vi "Add Alias_Alias and Alias Folder.vi"(8 "error in (no error)":errorcluster, 9 "Alias Settings":T1, 11 "SysDef Ref":T2) -> (0 "error out":errorcluster, 3 "SysDef Ref Out":T2)   [LabVIEW 2019, in "Simple SysDef API.lvlib"]
uses:
  <userlib>/SimpleSysDef/Simple SysDef API.lvlib
  <userlib>/SimpleSysDef/_SubVIs/System Definition Reference.ctl
  NationalInstruments.VeriStand.SystemDefinitionAPI
  <userlib>/SimpleSysDef/_SubVIs/Add Alias_Alias Settings.ctl
  <userlib>/SimpleSysDef/_SubVIs/Add Folder_Settings.ctl
  <userlib>/SimpleSysDef/_SubVIs/Add Alias Folder.vi
  <userlib>/SimpleSysDef/_SubVIs/Add Alias.vi
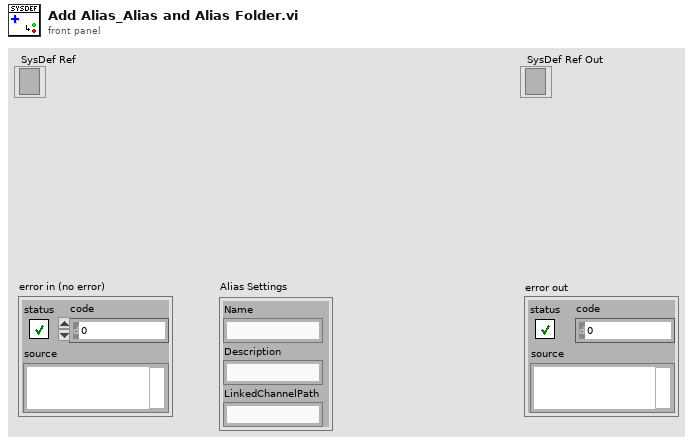
[diagram p1: front panel]
types:
  T1 = typedef "Simple SysDef API.lvlib/Add Alias_Alias Settings.ctl" = cluster{"Name":string, "Description":string, "LinkedChannelPath":string}
  T2 = typedef "Simple SysDef API.lvlib/System Definition Reference.ctl" = refnum<k24>
  T3 = typedef "Simple SysDef API.lvlib/Add Folder_Settings.ctl" = cluster{"Name":string, "Description":string}
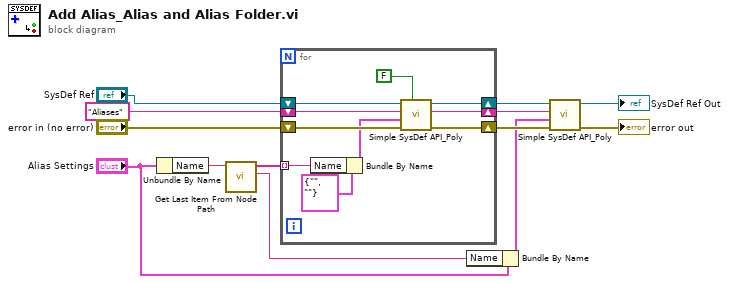
[diagram p0: block diagram]
diagram:
  n1 = Unbundle By Name("Alias Settings") -> ("Name"=w3:string)
  n2 = call <userlib>:"Get Last Item From Node Path.vi"("Name"=w3) -> ("Last Item"=w1:string, "First Items"=w2:string[])  [unwired: 9 in]
  n3 = for {
    shift-right: [w22] -> w12
    shift-left: "error in (no error)" -> [w19]
    shift-right: [w21] -> w11
    shift-left: "Aliases" ("Base Node Path") -> [w18]
    shift-right: [w23] -> w13
    shift-left: "SysDef Ref" -> [w20]
    tunnel: w2 -> [w16] mode=indexing
    n4 = Bundle By Name(cluster=T3 {"Name"="", "Description"=""} ("Alias Folder Settings"), "Name"=w16) -> (w15:T3)
    n5 = call-poly <userlib>:"Simple SysDef API_Poly.vi"("Overwrite Existing?"=FALSE, "error in (no error)"=w19, "Alias Folder Settings"=w15, "Base Node Path"=w18, "SysDef Ref"=w20) -> ("error out"=w22:errorcluster, "New Node Path"=w21:string, "SysDef Ref Out"=w23:T2)  [unwired: 4 in]
  }
  n6 = Bundle By Name(cluster="Alias Settings", "Name"=w1) -> (w4:T1)
  n7 = call-poly <userlib>:"Simple SysDef API_Poly.vi"("error in (no error)"=w12, "Alias Settings"=w4, "Base Node Path"=w11, "SysDef Ref"=w13) -> ("error out"=→"error out":errorcluster, "SysDef Ref Out"=→"SysDef Ref Out":T2)  [unwired: 5 in, 1 out]
